vi "DrivePathPlanPreview.vi"() -> (1 "LeftTrajectory":T2[](array[typedef]), 2 "RightTrajectory":T2[](array[typedef]), 3 "Go":bool)   [LabVIEW 2017]
uses:
  Pathfinder/Pathfinder-LabVIEW/Pathfinder-Lib/VIs/Waypoint.ctl
  Autonomous/PathPlannerSupport/TypeDefs/DrivePathfinderParams.ctl
  <vilib>/Rock Robotics/WPI/ThirdParty/Phoenix-LabVIEW/Motor Controller/Controls/CTRE_Phoenix_MotorControl_TrajectoryPointTimeDur.ctl
  Pathfinder/Pathfinder-LabVIEW/Pathfinder-Lib/VIs/Segment.ctl
  ArgosLib/Signal Processing/TypeDefs/EdgeDetector_Type.ctl
  General/MotionProfiling/TypeDefs/TrajectoryPoint.ctl
  ArgosLib/ArgosLib.lvlib
  Pathfinder/Pathfinder-LabVIEW/Pathfinder-Lib/Pathfinder.lvlib
panel:
  out "Left Drive Graph":T1(graph)
  out "Right Drive Graph":T1(graph)
  in  "DrivePathPlanParams":T3={"max_velocity (in/s)"=100.0, "max_acceleration (in/s^2)"=80.0, "max_jerk (in/s^3)"=100.0, "dt(ms)"=40, "sample_count"=1000, "wheelbase_width (in)"=25.0} {"dt(ms)" items=["TrajectoryDuration_0ms"=0, "TrajectoryDuration_5ms"=5, "TrajectoryDuration_10ms"=10, "TrajectoryDuration_20ms"=20, "TrajectoryDuration_30ms"=30, "TrajectoryDuration_40ms"=40, "TrajectoryDuration_50ms"=50, "TrajectoryDuration_100ms"=100]}
  in  "path":T5[](array[typedef])=[{"x"=19.5, "y"=160.0, "angle"=0.0}, {"x"=126.0, "y"=116.0, "angle"=0.0}]
  in  "Preview?":bool
  in  "Send Path Plan":bool
  in  "Reverse Direction":bool
  # "Center Start: (19.5, 160)\nLeft Switch: (120.5, 216)\nRight Switch: (126, 116)"
  # "Wheelbase: 25\"\nLength (bumper to bumper): 39\"\nWidth (bumper to bumper): 34\""
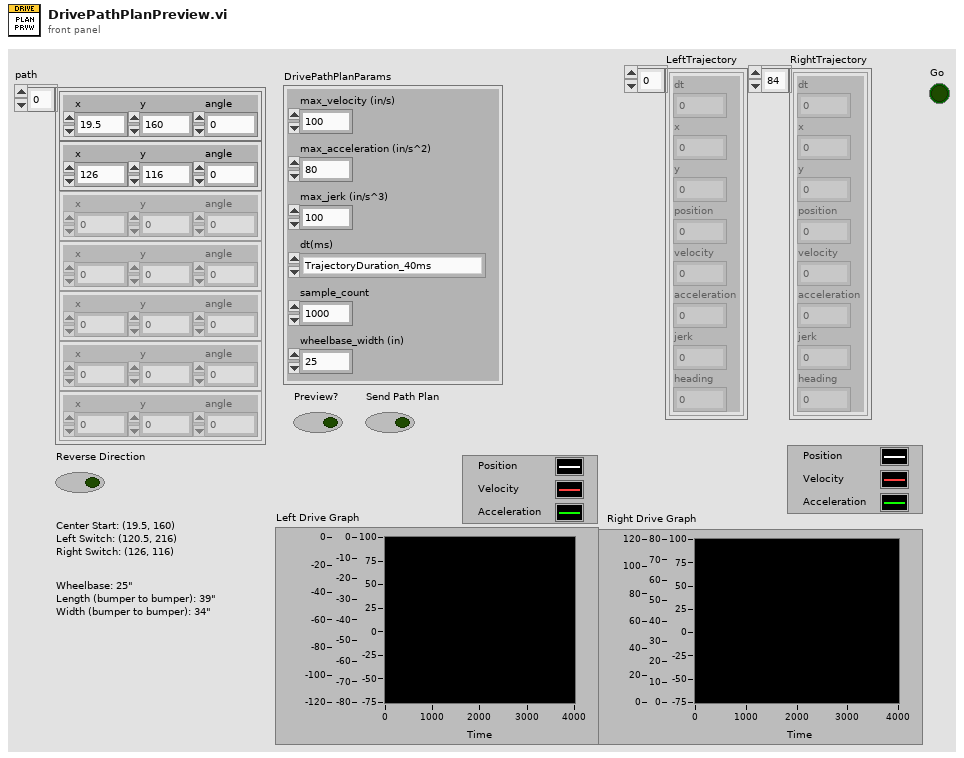
[diagram p1: front panel]
types:
  T1 = cluster{dbl, "Trajectory Point Interval (ms)":i32, dbl[][]}
  T2 = typedef "Pathfinder.lvlib/Segment.ctl" = cluster{"dt":dbl, "x":dbl, "y":dbl, "position":dbl, "velocity":dbl, "acceleration":dbl, "jerk":dbl, "heading":dbl}
  T3 = typedef "DrivePathfinderParams.ctl" = cluster{"max_velocity (in/s)":dbl, "max_acceleration (in/s^2)":dbl, "max_jerk (in/s^3)":dbl, "dt(ms)":T4, "sample_count":i32, "wheelbase_width (in)":dbl}
  T4 = typedef "CTRE_Phoenix_MotorControl_TrajectoryPointTimeDur.ctl" = i32
  T5 = typedef "Pathfinder.lvlib/Waypoint.ctl" = cluster{"x":dbl, "y":dbl, "angle":dbl}
  T6 = typedef "ArgosLib.lvlib/EdgeDetector_Type.ctl" = enum16{"RisingEdge", "FallingEdge", "Both"}
  T7 = typedef "TrajectoryPoint.ctl" = cluster{"Position ":dbl, "Velocity ":dbl, "Time (ms)":T4, "Last Point":bool}
  T8 = cluster{dbl, "Trajectory Point Interval (ms)":T4, dbl[][]}
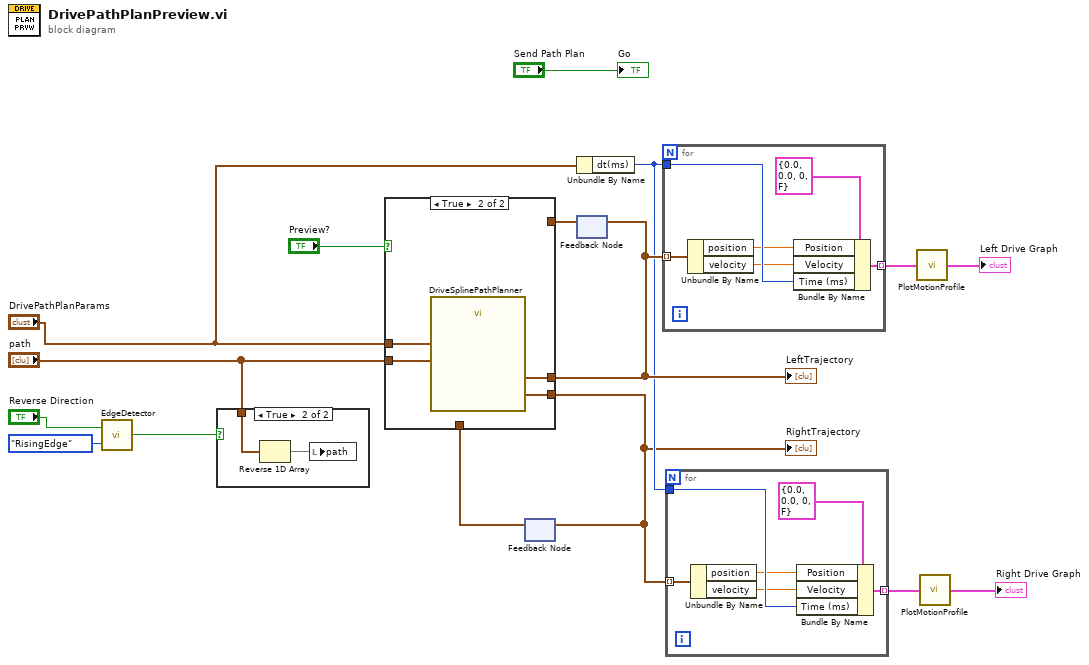
[diagram p0: block diagram]
diagram:
  n1 = call "EdgeDetector.vi"("DetectorType"=EdgeDetector_Type."RisingEdge", "Input"="Reverse Direction") -> ("Edge"=w16:bool)
  n2 = case shown="True" w16 {
    tunnel: "path" -> [_ w18]
    frame False {
    }
    frame True {
      n3 = Reverse 1D Array(array=w18) -> (reversed array=w17:T5[])
      n4 = local write "path"(w17) -> ()
    }
  }
  n5 = feedback #1() -> (w11:T2[])  [unwired: 1 in]
  n6 = Unbundle By Name("DrivePathPlanParams") -> ("dt(ms)"=w3:T4)
  n7 = feedback #2() -> (w10:T2[])  [unwired: 1 in]
  n8 = case shown="True" "Preview?" {
    tunnel: [w19 w23] -> w8
    tunnel: [w20 w24] -> w2
    tunnel: w11 -> [w20 _]
    tunnel: w10 -> [w19 _]
    tunnel: "path" -> [_ w22]
    tunnel: "DrivePathPlanParams" -> [_ w21]
    frame False {
    }
    frame True {
      n9 = call "DriveSplinePathPlanner.vi"("DrivePathPlanParams"=w21, "path"=w22) -> ("RightTrajectory"=w24:T2[], "LeftTrajectory"=w23:T2[])  [unwired: 1 in, 1 out]
    }
  }
  "LeftTrajectory" <- w8
  "RightTrajectory" <- w2
  n10 = feedback-in #1(w2) -> ()
  n11 = feedback-in #2(w8) -> ()
  n12 = for {
    tunnel: w8 -> [w27] mode=indexing
    tunnel: [w29] -> w6 mode=indexing
    tunnel: w3 -> [w28]
    n13 = Unbundle By Name(w27) -> ("position"=w26:dbl, "velocity"=w25:dbl)
    n14 = Bundle By Name(cluster=T7 {"Position "=0.0, "Velocity "=0.0, "Time (ms)"=0, "Last Point"=FALSE} ("trajectory point"), "Position"=w26, "Velocity"=w25, "Time (ms)"=w28) -> (w29:T7)
  }
  n15 = for {
    tunnel: w2 -> [w33] mode=indexing
    tunnel: [w35] -> w4 mode=indexing
    tunnel: w3 -> [w34]
    n16 = Unbundle By Name(w33) -> ("position"=w32:dbl, "velocity"=w31:dbl)
    n17 = Bundle By Name(cluster=T7 {"Position "=0.0, "Velocity "=0.0, "Time (ms)"=0, "Last Point"=FALSE} ("trajectory point"), "Position"=w32, "Velocity"=w31, "Time (ms)"=w34) -> (w35:T7)
  }
  n18 = call "PlotMotionProfile.vi"("Trajectory Points"=w6) -> ("MotionProfileGraph"=→"Left Drive Graph":T8)
  n19 = call "PlotMotionProfile.vi"("Trajectory Points"=w4) -> ("MotionProfileGraph"=→"Right Drive Graph":T8)
  "Go" <- "Send Path Plan"
